vi "RTS Read Latest Pattern Data.vi"(8 "Error In":errorcluster, 10 "All Door Opener Ctrl in":T1={"Station 1"={"Station Freezer"={"Time Count (s)"=0.0, "Status"="", "Door State"=FALSE, "Delay"=FALSE, "Chamber 1-1"=[], "Index"=0, "Delay Status"=""}, "Station Cab"={"Time Count (s)"=0.0, "Status"="", "Door State"=FALSE, "Delay"=FALSE, "Chamber 1-1"=[], "Index"=0, "Delay Status"=""}, "Station Slide"={"Time Count (s)"=0.0, "Status"="", "Door State"=FALSE, "Delay"=FALSE, "Chamber 1-1"=[], "Index"=0, "Delay Status"=""}, "1st Complete"=FALSE, "2nd Complete"=FALSE, "3rd Complete"=FALSE}, "Station 2"={"Station Freezer"={"Time Count (s)"=0.0, "Status"="", "Door State"=FALSE, "Delay"=FALSE, "Chamber 1-1"=[], "Index"=0, "Delay Status"=""}, "Station Cab"={"Time Count (s)"=0.0, "Status"="", "Door State"=FALSE, "Delay"=FALSE, "Chamber 1-1"=[], "Index"=0, "Delay Status"=""}, "Station Slide"={"Time Count (s)"=0.0, "Status"="", "Door State"=FALSE, "Delay"=FALSE, "Chamber 1-1"=[], "Index"=0, "Delay Status"=""}, "1st Complete"=FALSE, "2nd Complete"=FALSE, "3rd Complete"=FALSE}, "Station 3"={"Station Freezer"={"Time Count (s)"=0.0, "Status"="", "Door State"=FALSE, "Delay"=FALSE, "Chamber 1-1"=[], "Index"=0, "Delay Status"=""}, "Station Cab"={"Time Count (s)"=0.0, "Status"="", "Door State"=FALSE, "Delay"=FALSE, "Chamber 1-1"=[], "Index"=0, "Delay Status"=""}, "Station Slide"={"Time Count (s)"=0.0, "Status"="", "Door State"=FALSE, "Delay"=FALSE, "Chamber 1-1"=[], "Index"=0, "Delay Status"=""}, "1st Complete"=FALSE, "2nd Complete"=FALSE, "3rd Complete"=FALSE}, "Station 4"={"Station Freezer"={"Time Count (s)"=0.0, "Status"="", "Door State"=FALSE, "Delay"=FALSE, "Chamber 1-1"=[], "Index"=0, "Delay Status"=""}, "Station Cab"={"Time Count (s)"=0.0, "Status"="", "Door State"=FALSE, "Delay"=FALSE, "Chamber 1-1"=[], "Index"=0, "Delay Status"=""}, "Station Slide"={"Time Count (s)"=0.0, "Status"="", "Door State"=FALSE, "Delay"=FALSE, "Chamber 1-1"=[], "Index"=0, "Delay Status"=""}, "1st Complete"=FALSE, "2nd Complete"=FALSE, "3rd Complete"=FALSE}, "Station 5"={"Station Freezer"={"Time Count (s)"=0.0, "Status"="", "Door State"=FALSE, "Delay"=TRUE, "Chamber 1-1"=[], "Index"=0, "Delay Status"=""}, "Station Cab"={"Time Count (s)"=0.0, "Status"="", "Door State"=FALSE, "Delay"=TRUE, "Chamber 1-1"=[], "Index"=0, "Delay Status"=""}, "Station Slide"={"Time Count (s)"=0.0, "Status"="", "Door State"=FALSE, "Delay"=TRUE, "Chamber 1-1"=[], "Index"=0, "Delay Status"=""}, "1st Complete"=FALSE, "2nd Complete"=FALSE, "3rd Complete"=FALSE}, "Station 6"={"Station Freezer"={"Time Count (s)"=0.0, "Status"="", "Door State"=FALSE, "Delay"=TRUE, "Chamber 1-1"=[], "Index"=0, "Delay Status"=""}, "Station Cab"={"Time Count (s)"=0.0, "Status"="", "Door State"=FALSE, "Delay"=TRUE, "Chamber 1-1"=[], "Index"=0, "Delay Status"=""}, "Station Slide"={"Time Count (s)"=0.0, "Status"="", "Door State"=FALSE, "Delay"=TRUE, "Chamber 1-1"=[], "Index"=0, "Delay Status"=""}, "1st Complete"=FALSE, "2nd Complete"=FALSE, "3rd Complete"=FALSE}, "Station 7"={"Station Freezer"={"Time Count (s)"=0.0, "Status"="", "Door State"=FALSE, "Delay"=TRUE, "Chamber 1-1"=[], "Index"=0, "Delay Status"=""}, "Station Cab"={"Time Count (s)"=0.0, "Status"="", "Door State"=FALSE, "Delay"=TRUE, "Chamber 1-1"=[], "Index"=0, "Delay Status"=""}, "Station Slide"={"Time Count (s)"=0.0, "Status"="", "Door State"=FALSE, "Delay"=TRUE, "Chamber 1-1"=[], "Index"=0, "Delay Status"=""}, "1st Complete"=FALSE, "2nd Complete"=FALSE, "3rd Complete"=FALSE}, "Station 8"={"Station Freezer"={"Time Count (s)"=0.0, "Status"="", "Door State"=FALSE, "Delay"=TRUE, "Chamber 1-1"=[], "Index"=0, "Delay Status"=""}, "Station Cab"={"Time Count (s)"=0.0, "Status"="", "Door State"=FALSE, "Delay"=TRUE, "Chamber 1-1"=[], "Index"=0, "Delay Status"=""}, "Station Slide"={"Time Count (s)"=0.0, "Status"="", "Door State"=FALSE, "Delay"=TRUE, "Chamber 1-1"=[], "Index"=0, "Delay Status"=""}, "1st Complete"=FALSE, "2nd Complete"=FALSE, "3rd Complete"=FALSE}} {"Station 8"."Station Slide"."Chamber 1-1"."Start Time" format="%<%X\n%x>T"; "Station 8"."Station Slide"."Chamber 1-1"."End Time" format="%<%X\n%x>T"; "Station 8"."Station Slide"."Time Count (s)" format="%.2f"; "Station 8"."Station Cab"."Chamber 1-1"."Start Time" format="%<%X\n%x>T"; "Station 8"."Station Cab"."Chamber 1-1"."End Time" format="%<%X\n%x>T"; "Station 8"."Station Cab"."Time Count (s)" format="%.2f"; "Station 8"."Station Freezer"."Chamber 1-1"."Start Time" format="%<%X\n%x>T"; "Station 8"."Station Freezer"."Chamber 1-1"."End Time" format="%<%X\n%x>T"; "Station 8"."Station Freezer"."Time Count (s)" format="%.2f"; "Station 7"."Station Slide"."Chamber 1-1"."Start Time" format="%<%X\n%x>T"; "Station 7"."Station Slide"."Chamber 1-1"."End Time" format="%<%X\n%x>T"; "Station 7"."Station Slide"."Time Count (s)" format="%.2f"; "Station 7"."Station Cab"."Chamber 1-1"."Start Time" format="%<%X\n%x>T"; "Station 7"."Station Cab"."Chamber 1-1"."End Time" format="%<%X\n%x>T"; "Station 7"."Station Cab"."Time Count (s)" format="%.2f"; "Station 7"."Station Freezer"."Chamber 1-1"."Start Time" format="%<%X\n%x>T"; "Station 7"."Station Freezer"."Chamber 1-1"."End Time" format="%<%X\n%x>T"; "Station 7"."Station Freezer"."Time Count (s)" format="%.2f"; "Station 6"."Station Slide"."Chamber 1-1"."Start Time" format="%<%X\n%x>T"; "Station 6"."Station Slide"."Chamber 1-1"."End Time" format="%<%X\n%x>T"; "Station 6"."Station Slide"."Time Count (s)" format="%.2f"; "Station 6"."Station Cab"."Chamber 1-1"."Start Time" format="%<%X\n%x>T"; "Station 6"."Station Cab"."Chamber 1-1"."End Time" format="%<%X\n%x>T"; "Station 6"."Station Cab"."Time Count (s)" format="%.2f"; "Station 6"."Station Freezer"."Chamber 1-1"."Start Time" format="%<%X\n%x>T"; "Station 6"."Station Freezer"."Chamber 1-1"."End Time" format="%<%X\n%x>T"; "Station 6"."Station Freezer"."Time Count (s)" format="%.2f"; "Station 5"."Station Slide"."Chamber 1-1"."Start Time" format="%<%X\n%x>T"; "Station 5"."Station Slide"."Chamber 1-1"."End Time" format="%<%X\n%x>T"; "Station 5"."Station Slide"."Time Count (s)" format="%.2f"; "Station 5"."Station Cab"."Chamber 1-1"."Start Time" format="%<%X\n%x>T"; "Station 5"."Station Cab"."Chamber 1-1"."End Time" format="%<%X\n%x>T"; "Station 5"."Station Cab"."Time Count (s)" format="%.2f"; "Station 5"."Station Freezer"."Chamber 1-1"."Start Time" format="%<%X\n%x>T"; "Station 5"."Station Freezer"."Chamber 1-1"."End Time" format="%<%X\n%x>T"; "Station 5"."Station Freezer"."Time Count (s)" format="%.2f"; "Station 4"."Station Slide"."Chamber 1-1"."Start Time" format="%<%X\n%x>T"; "Station 4"."Station Slide"."Chamber 1-1"."End Time" format="%<%X\n%x>T"; "Station 4"."Station Slide"."Time Count (s)" format="%.2f"; "Station 4"."Station Cab"."Chamber 1-1"."Start Time" format="%<%X\n%x>T"; "Station 4"."Station Cab"."Chamber 1-1"."End Time" format="%<%X\n%x>T"; "Station 4"."Station Cab"."Time Count (s)" format="%.2f"; "Station 4"."Station Freezer"."Chamber 1-1"."Start Time" format="%<%X\n%x>T"; "Station 4"."Station Freezer"."Chamber 1-1"."End Time" format="%<%X\n%x>T"; "Station 4"."Station Freezer"."Time Count (s)" format="%.2f"; "Station 3"."Station Slide"."Chamber 1-1"."Start Time" format="%<%X\n%x>T"; "Station 3"."Station Slide"."Chamber 1-1"."End Time" format="%<%X\n%x>T"; "Station 3"."Station Slide"."Time Count (s)" format="%.2f"; "Station 3"."Station Cab"."Chamber 1-1"."Start Time" format="%<%X\n%x>T"; "Station 3"."Station Cab"."Chamber 1-1"."End Time" format="%<%X\n%x>T"; "Station 3"."Station Cab"."Time Count (s)" format="%.2f"; "Station 3"."Station Freezer"."Chamber 1-1"."Start Time" format="%<%X\n%x>T"; "Station 3"."Station Freezer"."Chamber 1-1"."End Time" format="%<%X\n%x>T"; "Station 3"."Station Freezer"."Time Count (s)" format="%.2f"; "Station 2"."Station Slide"."Chamber 1-1"."Start Time" format="%<%X\n%x>T"; "Station 2"."Station Slide"."Chamber 1-1"."End Time" format="%<%X\n%x>T"; "Station 2"."Station Slide"."Time Count (s)" format="%.2f"; "Station 2"."Station Cab"."Chamber 1-1"."Start Time" format="%<%X\n%x>T"; "Station 2"."Station Cab"."Chamber 1-1"."End Time" format="%<%X\n%x>T"; "Station 2"."Station Cab"."Time Count (s)" format="%.2f"; "Station 2"."Station Freezer"."Chamber 1-1"."Start Time" format="%<%X\n%x>T"; "Station 2"."Station Freezer"."Chamber 1-1"."End Time" format="%<%X\n%x>T"; "Station 2"."Station Freezer"."Time Count (s)" format="%.2f"; "Station 1"."Station Slide"."Chamber 1-1"."Start Time" format="%<%X\n%x>T"; "Station 1"."Station Slide"."Chamber 1-1"."End Time" format="%<%X\n%x>T"; "Station 1"."Station Slide"."Time Count (s)" format="%.2f"; "Station 1"."Station Cab"."Chamber 1-1"."Start Time" format="%<%X\n%x>T"; "Station 1"."Station Cab"."Chamber 1-1"."End Time" format="%<%X\n%x>T"; "Station 1"."Station Cab"."Time Count (s)" format="%.2f"; "Station 1"."Station Freezer"."Chamber 1-1"."Start Time" format="%<%X\n%x>T"; "Station 1"."Station Freezer"."Chamber 1-1"."End Time" format="%<%X\n%x>T"; "Station 1"."Station Freezer"."Time Count (s)" format="%.2f"}, 11 "RTS Config Setup":T7) -> (0 "Error Out":errorcluster, 3 "All Door Opener Ctrl out":T1 {"Station 8"."Station Slide"."Chamber 1-1"."Start Time" format="%<%X\n%x>T"; "Station 8"."Station Slide"."Chamber 1-1"."End Time" format="%<%X\n%x>T"; "Station 8"."Station Slide"."Time Count (s)" format="%.2f"; "Station 8"."Station Cab"."Chamber 1-1"."Start Time" format="%<%X\n%x>T"; "Station 8"."Station Cab"."Chamber 1-1"."End Time" format="%<%X\n%x>T"; "Station 8"."Station Cab"."Time Count (s)" format="%.2f"; "Station 8"."Station Freezer"."Chamber 1-1"."Start Time" format="%<%X\n%x>T"; "Station 8"."Station Freezer"."Chamber 1-1"."End Time" format="%<%X\n%x>T"; "Station 8"."Station Freezer"."Time Count (s)" format="%.2f"; "Station 7"."Station Slide"."Chamber 1-1"."Start Time" format="%<%X\n%x>T"; "Station 7"."Station Slide"."Chamber 1-1"."End Time" format="%<%X\n%x>T"; "Station 7"."Station Slide"."Time Count (s)" format="%.2f"; "Station 7"."Station Cab"."Chamber 1-1"."Start Time" format="%<%X\n%x>T"; "Station 7"."Station Cab"."Chamber 1-1"."End Time" format="%<%X\n%x>T"; "Station 7"."Station Cab"."Time Count (s)" format="%.2f"; "Station 7"."Station Freezer"."Chamber 1-1"."Start Time" format="%<%X\n%x>T"; "Station 7"."Station Freezer"."Chamber 1-1"."End Time" format="%<%X\n%x>T"; "Station 7"."Station Freezer"."Time Count (s)" format="%.2f"; "Station 6"."Station Slide"."Chamber 1-1"."Start Time" format="%<%X\n%x>T"; "Station 6"."Station Slide"."Chamber 1-1"."End Time" format="%<%X\n%x>T"; "Station 6"."Station Slide"."Time Count (s)" format="%.2f"; "Station 6"."Station Cab"."Chamber 1-1"."Start Time" format="%<%X\n%x>T"; "Station 6"."Station Cab"."Chamber 1-1"."End Time" format="%<%X\n%x>T"; "Station 6"."Station Cab"."Time Count (s)" format="%.2f"; "Station 6"."Station Freezer"."Chamber 1-1"."Start Time" format="%<%X\n%x>T"; "Station 6"."Station Freezer"."Chamber 1-1"."End Time" format="%<%X\n%x>T"; "Station 6"."Station Freezer"."Time Count (s)" format="%.2f"; "Station 5"."Station Slide"."Chamber 1-1"."Start Time" format="%<%X\n%x>T"; "Station 5"."Station Slide"."Chamber 1-1"."End Time" format="%<%X\n%x>T"; "Station 5"."Station Slide"."Time Count (s)" format="%.2f"; "Station 5"."Station Cab"."Chamber 1-1"."Start Time" format="%<%X\n%x>T"; "Station 5"."Station Cab"."Chamber 1-1"."End Time" format="%<%X\n%x>T"; "Station 5"."Station Cab"."Time Count (s)" format="%.2f"; "Station 5"."Station Freezer"."Chamber 1-1"."Start Time" format="%<%X\n%x>T"; "Station 5"."Station Freezer"."Chamber 1-1"."End Time" format="%<%X\n%x>T"; "Station 5"."Station Freezer"."Time Count (s)" format="%.2f"; "Station 4"."Station Slide"."Chamber 1-1"."Start Time" format="%<%X\n%x>T"; "Station 4"."Station Slide"."Chamber 1-1"."End Time" format="%<%X\n%x>T"; "Station 4"."Station Slide"."Time Count (s)" format="%.2f"; "Station 4"."Station Cab"."Chamber 1-1"."Start Time" format="%<%X\n%x>T"; "Station 4"."Station Cab"."Chamber 1-1"."End Time" format="%<%X\n%x>T"; "Station 4"."Station Cab"."Time Count (s)" format="%.2f"; "Station 4"."Station Freezer"."Chamber 1-1"."Start Time" format="%<%X\n%x>T"; "Station 4"."Station Freezer"."Chamber 1-1"."End Time" format="%<%X\n%x>T"; "Station 4"."Station Freezer"."Time Count (s)" format="%.2f"; "Station 3"."Station Slide"."Chamber 1-1"."Start Time" format="%<%X\n%x>T"; "Station 3"."Station Slide"."Chamber 1-1"."End Time" format="%<%X\n%x>T"; "Station 3"."Station Slide"."Time Count (s)" format="%.2f"; "Station 3"."Station Cab"."Chamber 1-1"."Start Time" format="%<%X\n%x>T"; "Station 3"."Station Cab"."Chamber 1-1"."End Time" format="%<%X\n%x>T"; "Station 3"."Station Cab"."Time Count (s)" format="%.2f"; "Station 3"."Station Freezer"."Chamber 1-1"."Start Time" format="%<%X\n%x>T"; "Station 3"."Station Freezer"."Chamber 1-1"."End Time" format="%<%X\n%x>T"; "Station 3"."Station Freezer"."Time Count (s)" format="%.2f"; "Station 2"."Station Slide"."Chamber 1-1"."Start Time" format="%<%X\n%x>T"; "Station 2"."Station Slide"."Chamber 1-1"."End Time" format="%<%X\n%x>T"; "Station 2"."Station Slide"."Time Count (s)" format="%.2f"; "Station 2"."Station Cab"."Chamber 1-1"."Start Time" format="%<%X\n%x>T"; "Station 2"."Station Cab"."Chamber 1-1"."End Time" format="%<%X\n%x>T"; "Station 2"."Station Cab"."Time Count (s)" format="%.2f"; "Station 2"."Station Freezer"."Chamber 1-1"."Start Time" format="%<%X\n%x>T"; "Station 2"."Station Freezer"."Chamber 1-1"."End Time" format="%<%X\n%x>T"; "Station 2"."Station Freezer"."Time Count (s)" format="%.2f"; "Station 1"."Station Slide"."Chamber 1-1"."Start Time" format="%<%X\n%x>T"; "Station 1"."Station Slide"."Chamber 1-1"."End Time" format="%<%X\n%x>T"; "Station 1"."Station Slide"."Time Count (s)" format="%.2f"; "Station 1"."Station Cab"."Chamber 1-1"."Start Time" format="%<%X\n%x>T"; "Station 1"."Station Cab"."Chamber 1-1"."End Time" format="%<%X\n%x>T"; "Station 1"."Station Cab"."Time Count (s)" format="%.2f"; "Station 1"."Station Freezer"."Chamber 1-1"."Start Time" format="%<%X\n%x>T"; "Station 1"."Station Freezer"."Chamber 1-1"."End Time" format="%<%X\n%x>T"; "Station 1"."Station Freezer"."Time Count (s)" format="%.2f"})   [LabVIEW 2016]
uses:
  Type Definitions/RTS All Station Door Opener Ctrl.ctl
  Type Definitions/RTS Station Relay Ops.ctl
  Type Definitions/RTS Door Opener Indicator.ctl
  Type Definitions/RTS Door Ops Client.ctl
  Type Definitions/RTS Door Opening Schedule.ctl
  Type Definitions/RTS Door Ops Sequence.ctl
  Type Definitions/RTS Configuration Setup.ctl
  Type Definitions/RTS Wago Config.ctl
  Type Definitions/RTS APLUS Config.ctl
  Type Definitions/RTS Yokogawa MX Config.ctl
  Type Definitions/RTS Replay Server Control.ctl
  Type Definitions/RTS Server Configuration.ctl
  Type Definitions/RTS Station Settions TCP Comms.ctl
  Type Definitions/RTS Chamber Save Status.ctl
  Type Definitions/RTS Test Pattern.ctl
panel:
  # "Chamber Conditions:"
  # "Chamber Conditions:"
  # "Chamber Conditions:"
  # "Chamber Conditions:"
  # "Chamber Conditions:"
  # "Chamber Conditions:"
  # "Chamber Conditions:"
  # "Chamber Conditions:"
  # "Chamber Conditions:"
  # "Chamber Conditions:"
  # "Chamber Conditions:"
  # "Chamber Conditions:"
  # "Chamber Conditions:"
  # "Chamber Conditions:"
  # "Chamber Conditions:"
  # "Chamber Conditions:"
  # "Chamber Conditions:"
  # "Chamber Conditions:"
  # "Chamber Conditions:"
  # "Chamber Conditions:"
  # "Chamber Conditions:"
  # "Chamber Conditions:"
  # "Chamber Conditions:"
  # "Chamber Conditions:"
  # "Chamber Conditions:"
  # "Chamber Conditions:"
  # "Chamber Conditions:"
  # "Chamber Conditions:"
  # "Chamber Conditions:"
  # "Chamber Conditions:"
  # "Chamber Conditions:"
  # "Chamber Conditions:"
  # "Chamber Conditions:"
  # "Chamber Conditions:"
  # "Chamber Conditions:"
  # "Chamber Conditions:"
  # "Chamber Conditions:"
  # "Chamber Conditions:"
  # "Chamber Conditions:"
  # "Chamber Conditions:"
  # "Chamber Conditions:"
  # "Chamber Conditions:"
  # "Chamber Conditions:"
  # "Chamber Conditions:"
  # "Chamber Conditions:"
  # "Chamber Conditions:"
  # "Chamber Conditions:"
  # "Chamber Conditions:"
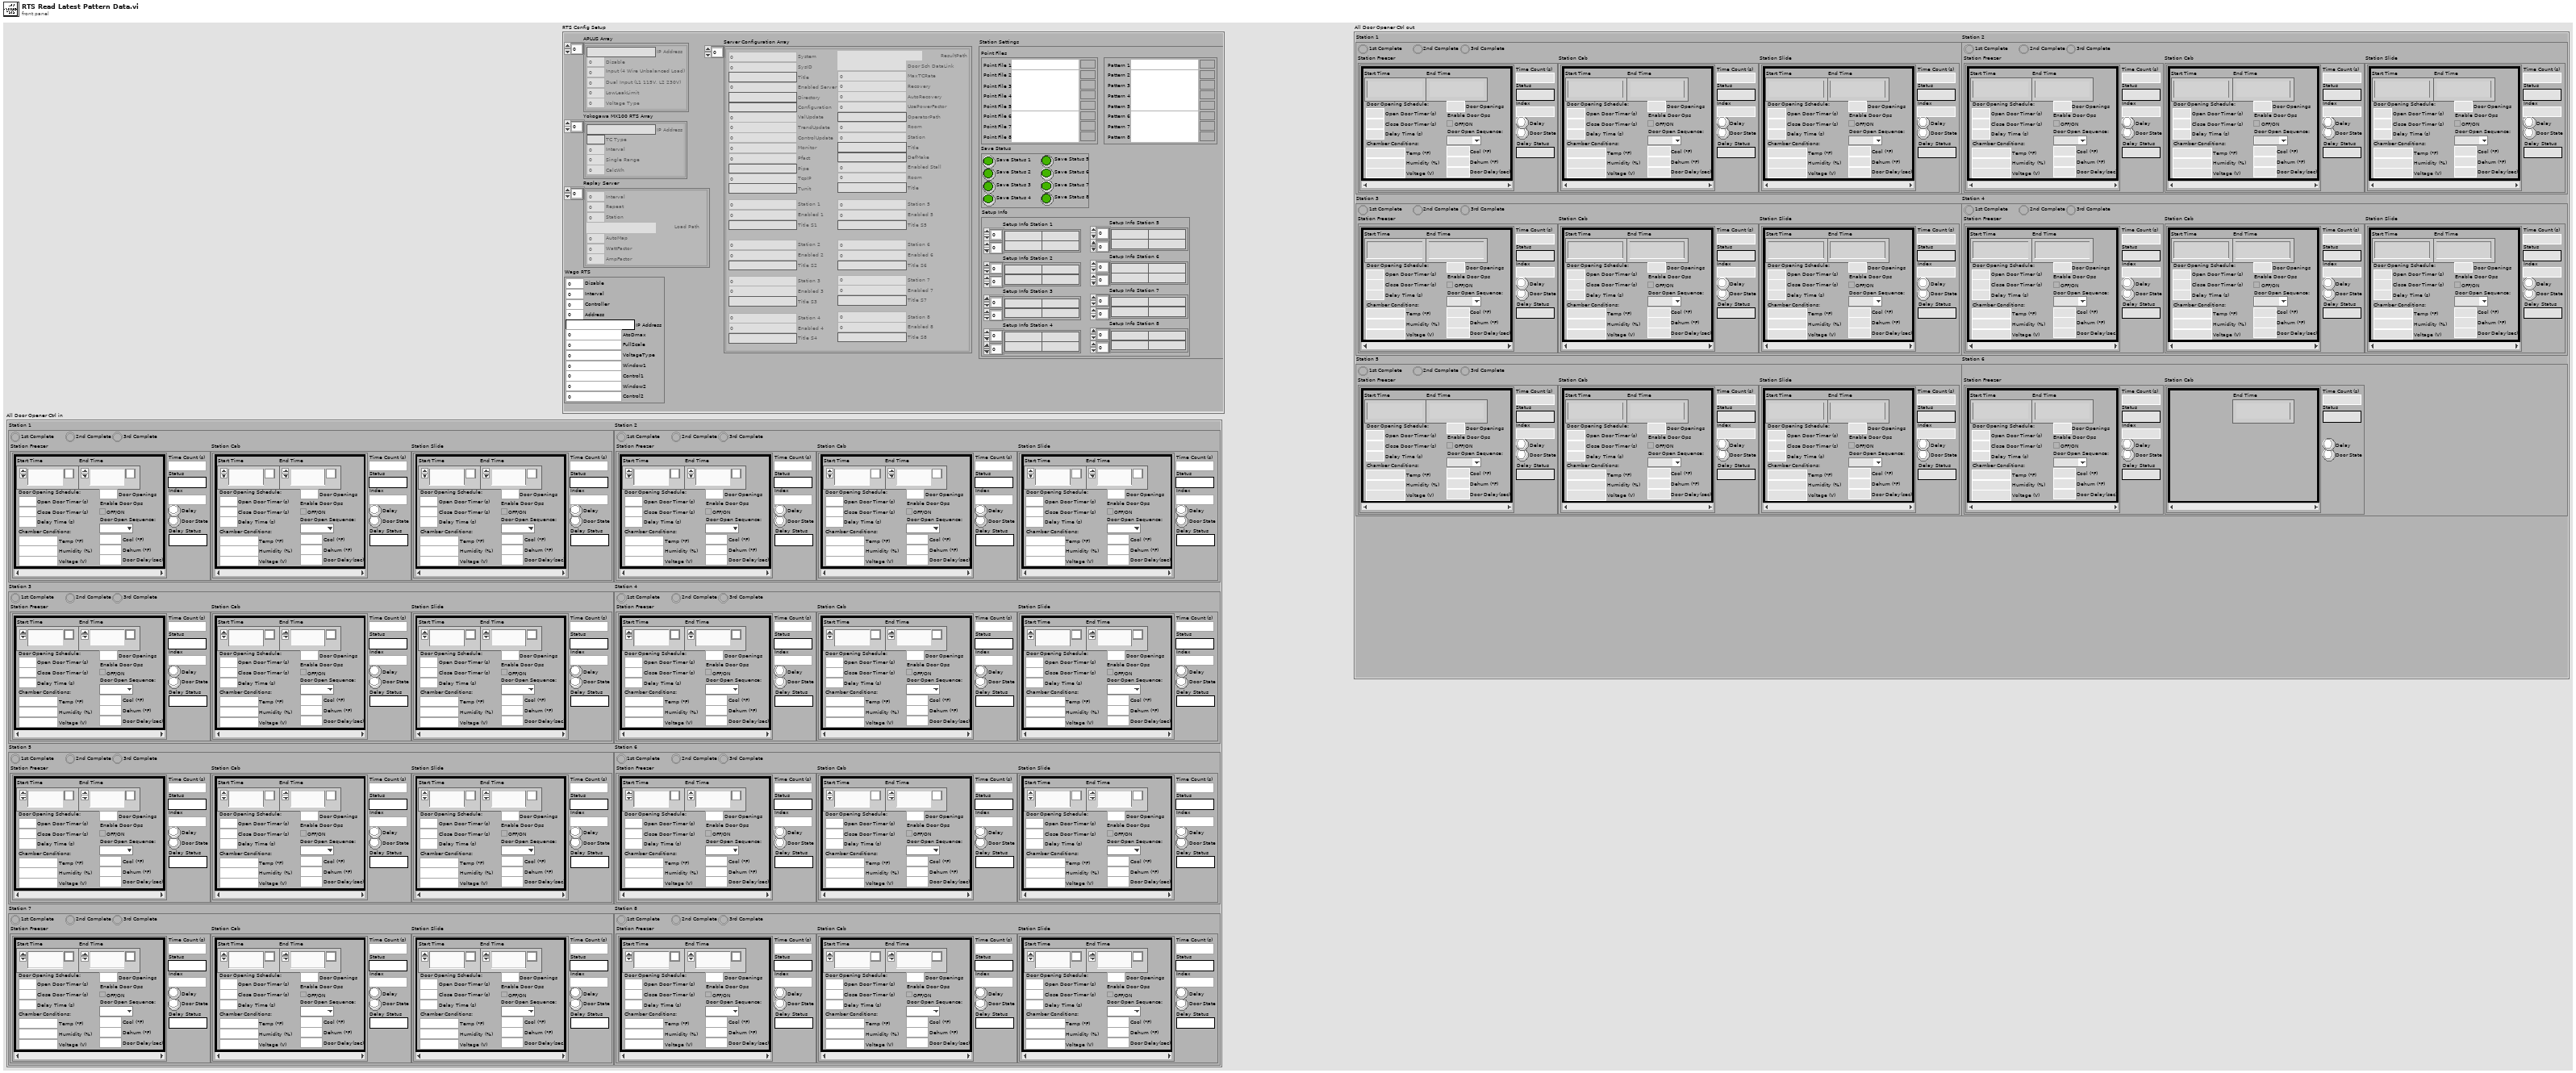
[diagram p1: front panel]
types:
  T1 = typedef "RTS All Station Door Opener Ctrl.ctl" = cluster{"Station 1":T2, "Station 2":T2, "Station 3":T2, "Station 4":T2, "Station 5":T2, "Station 6":T2, "Station 7":T2, "Station 8":T2}
  T2 = typedef "RTS Station Relay Ops.ctl" = cluster{"Station Freezer":T3, "Station Cab":T3, "Station Slide":T3, "1st Complete":bool, "2nd Complete":bool, "3rd Complete":bool}
  T3 = typedef "RTS Door Opener Indicator.ctl" = cluster{"Time Count (s)":dbl, "Status":string, "Door State":bool, "Delay":bool, "Chamber 1-1":T4[], "Index":i32, "Delay Status":string}
  T4 = typedef "RTS Door Ops Client.ctl" = cluster{"End Time":timestamp, "Start Time":timestamp, "Door Opening Schedule:":T5, "Enable Door Ops":bool, "Door Openings":u32, "Temp (°F)":dbl, "Humidity (%)":dbl, "Voltage (V)":dbl, "Door Open Sequence:":T6, "Door Delay(sec)":dbl, "Dehum (°F)":dbl, "Cool (°F)":dbl}
  T5 = typedef "RTS Door Opening Schedule.ctl" = cluster{"Open Door Timer (s)":dbl, "Delay Time (s)":dbl, "Close Door Timer (s)":dbl}
  T6 = typedef "RTS Door Ops Sequence.ctl" = enum16{"", "1st", "2nd", "3rd"}
  T7 = typedef "RTS Configuration Setup.ctl" = cluster{"Wago RTS":T8, "APLUS Array":T9[], "Yokogawa MX100 RTS Array":T10[], "Replay Server":T11[], "Server Configuration Array":T12[], "Station Settings":T13}
  T8 = typedef "RTS Wago Config.ctl" = cluster{"Disable":u16, "Interval":u16, "Controller":u16, "Address":u16, "IP Address":string, "AtoDmax":u16, "FullScale":u16, "VoltageType":u16, "Window1":u16, "Control1":u16, "Window2":u16, "Control2":u16}
  T9 = typedef "RTS APLUS Config.ctl" = cluster{"Disable":u16, "IP Address":string, "Input (4 Wire Unbalanced Load)":u16, "Dual Input (L1 115V, L2 230V)":u16, "LowLeakLimit":dbl, "Voltage Type":u16}
  T10 = typedef "RTS Yokogawa MX Config.ctl" = cluster{"IP Address":string, "TC Type":string, "Interval":u16, "Single Range":u16, "CalcWh":u16}
  T11 = typedef "RTS Replay Server Control.ctl" = cluster{"Interval":i16, "Repeat":u16, "Station":u16, "Load Path":path, "AutoMap":u16, "WattFactor":dbl, "AmpFactor":dbl}
  T12 = typedef "RTS Server Configuration.ctl" = cluster{"System":u16, "SysID":u16, "Title":string, "Enabled Server":u16, "Directory":string, "Configuration":string, "ValUpdate":u16, "TrendUpdate":u16, "ControlUpdate":u16, "Monitor":u16, "Pfact":u16, "Pipe":string, "TcpIP":u16, "Tunit":string, "ResultPath":path, "Door Sch DataLink":path, "MaxTCRate":u16, "Recovery":u16, "AutoRecovery":u16, "UsePowerFactor":u16, "OperatorPath":string, "Room":u16, "Station":u16, "Title":string, "DefMake":string, "Enabled Stall":u16, "Room":u16, "Title":string, "Station 1":u16, "Enabled 1":u16, "Station 2":u16, "Enabled 2":u16, "Station 3":u16, "Enabled 3":u16, "Station 4":u16, "Enabled 4":u16, "Station 5":u16, "Enabled 5":u16, "Station 6":u16, "Enabled 6":u16, "Station 7":u16, "Enabled 7":u16, "Station 8":u16, "Enabled 8":u16, "Title S1":string, "Title S2":string, "Title S3":string, "Title S5":string, "Title S6":string, "Title S7":string, "Title S8":string, "Title S4":string}
  T13 = typedef "RTS Station Settions TCP Comms.ctl" = cluster{"Point Files":cluster{"Point File 1":path, "Point File 2":path, "Point File 3":path, "Point File 4":path, "Point File 5":path, "Point File 6":path, "Point File 7":path, "Point File 8":path}, "Save Status":T14, "Setup Info":cluster{"Setup Info Station 1":string[][], "Setup Info Station 2":string[][], "Setup Info Station 3":string[][], "Setup Info Station 4":string[][], "Setup Info Station 5":string[][], "Setup Info Station 6":string[][], "Setup Info Station 7":string[][], "Setup Info Station 8":string[][]}, "Chamber Test Pattern":T15}
  T14 = typedef "RTS Chamber Save Status.ctl" = cluster{"Save Status 1":bool, "Save Status 2":bool, "Save Status 3":bool, "Save Status 4":bool, "Save Status 5":bool, "Save Status 6":bool, "Save Status 7":bool, "Save Status 8":bool}
  T15 = typedef "RTS Test Pattern.ctl" = cluster{" Pattern 1":path, "Pattern 2":path, "Pattern 3":path, "Pattern 4":path, "Pattern 5":path, "Pattern 6":path, "Pattern 7":path, "Pattern 8":path}
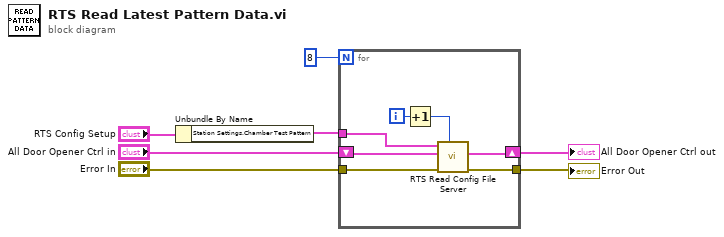
[diagram p0: block diagram]
diagram:
  n1 = Unbundle By Name("RTS Config Setup") -> ("Station Settings.Chamber Test Pattern"=w5:T15)
  n2 = for {
    N: 8 -> [_]
    tunnel: w5 -> [w11]
    shift-right: [w10] -> w4
    shift-left: "All Door Opener Ctrl in" -> [w14]
    tunnel: "Error In" -> [w8]
    tunnel: [w9] -> w2
    i -> [w13]
    n3 = Increment(x=w13) -> (x+1=w12:i32)
    n4 = call "RTS Read Config File Server.vi"("Station Number"=w12, "Error In"=w8, "All Door Opener Ctrl in"=w14, "Chamber Test Pattern"=w11) -> ("Error Out"=w9:errorcluster, "All Door Opener Ctrl Out"=w10:T1)  [unwired: 6 in]
  }
  "All Door Opener Ctrl out" <- w4
  "Error Out" <- w2
